vi "Package.vi"   [LabVIEW 2017]
doc: "Builds a VI package (vip) for this project for LabVIEW 2015."
uses:
  Support/LabVIEW Versions.ctl
panel:
  # "Overview: Builds a VI Package (vip) for LabVIEW versions >= 2015\nRequirements: LabVIEW 2015, VIPM Pro, VIPM API\nInstructions: Run this VI.\n\nThis VI attempts automate the building the VIP file for this add-on as much as possible. If VIPM Pro is not available, then the VIPM API will not work, and the building of the package must be done manually. This VI automates the following manual steps:\n\n1. Save the current project for LabVIEW 2015\n    a. From the Project Explorer window, select File->Save for Previous Version... A new dialog will appear.\n    b. Select \"15.0\" from the drop down menu.\n    c. Click \"Save...\". A new dialog will appear. Create a \"target\\15.0\" folder hierarchy in the root project folder (same location as the project file,    \n        .lvproj) if it does not already exist.\n    d. Click \"OK\". All of the contents of the project will be saved to LabVIEW 2015.\n2. Start LabVIEW 2015 and open the \"target\\15.0\\Eulogy.lvproj\" file created in Step 1. Do NOT open any file in the \"target\\15.0\" folder in any other \n    version of LabVIEW.\n3. Build all Source Distributions defined under \"Build Specifications\" tree item in the Project Explorer. A new \"target\\15.0\\builds\" folder will be \n    created with a sub-folder for each component.\n4. Expand the \"Configs\" virtual folder in the Project Explorer and double click on the \"Eulogy.vipb\" file. This will start the VIPM application.\n5. Click the \"Build\" icon near the top of the window for the Eulogy package specification. Do NOT alter any values, but ensure \"2015\" is selected at \n    the top right.\n6. Once the package is built, it will be available at \"target\\15.0\\packages\". \n\nNote, any version newer than LabVIEW 2015 can be used to run this VI and still have the package built for LabVIEW 2015, but the LabVIEW 2015 development environment must be installed.\n\nWhen this VI runs, it will automatically start LabVIEW 2015, build all of the components, start VIPM, build the package, then close both LabVIEW 2015 and VIPM. Another VI, \"Build Target.vi\" will run during this process. Do not abort or close the VI will running.\n\nThe oldest LabVIEW version possible for this add-on is LabVIEW 2015. LabVIEW 2015 introduced shortcut menu plugins, which are an integral usability component to this add-on. If the shortcut menu items are not needed, then the oldest version possible is LabVIEW 2013, which introduced custom bookmark managers. Similarly, custom bookmark managers are an integratl usability component for this add-on. All of the features and functionality are not possible with versions older than LabVIEW 2015."
types:
  T1 = typedef "LabVIEW Versions.ctl" = enum16{"2009", "2010", "2011", "2012", "2013", "2014", "2015", "2016", "2017", "2018"}
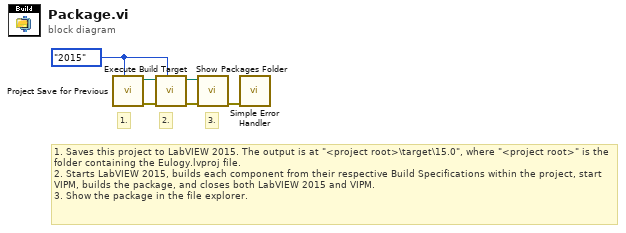
[diagram p0: block diagram]
diagram:
  w5 = LabVIEW_Versions."2015" ("LabVIEW Previous Version")
  # "3."
  # "2."
  # "1. Saves this project to LabVIEW 2015. The output is at \"<project root>\\target\\15.0\", where \"<project root>\" is the folder containing the Eulogy.lvproj file.\n2. Starts LabVIEW 2015, builds each component from their respective Build Specifications within the project, start VIPM, builds the package, and closes both LabVIEW 2015 and VIPM.\n3. Show the package in the file explorer."
  # "1."
  n1 = call "Project Save for Previous.vi"("LabVIEW Previous Version"=w5) -> ("Error Out"=w6:errorcluster, "Destination"=w2:path)  [unwired: 9 in]
  n2 = call "Execute Build Target.vi"("LabVIEW Previous Version"=w5, "Error In"=w6, "Target Project Root In"=w2) -> ("Error Out"=w3:errorcluster, "Target Project Root Out"=w1:path)  [unwired: 7 in]
  n3 = call "Show Packages Folder.vi"("Error In"=w3, "Target Project Root"=w1) -> ("Error Out"=w4:errorcluster)  [unwired: 9 in]
  n4 = call <vilib>:"Simple Error Handler.vi"("error in (no error)"=w4) -> ()  [unwired: 4 in, 5 out]
